vi "Test Save TGA (Memory).vi"(8 "error in (no error)":errorcluster) -> (0 "error out":errorcluster, 3 "Pass?":bool)   [LabVIEW 2020]
uses:
  <vilib>/picture/picture.llb/imagedata.ctl
  G-Image/Image IO/Polymorphic VIs/Save PNG Image (Memory).vi/23d07dd8-0246-46c8-8885-479f1b0fb2b3.vi
  G-Image/Private/Result To Error.vi
  G-Image/Private/Get Image Data.vi
  G-Image/Private/ARGB To RGBA.vi
  G-Image/Private/Depth To Number Channels.vi
  G-Image/Image Processing/Indexed Color To True Color Image.vi
  <vilib>/Utility/error.llb/Error Cluster From Error Code.vi
  G-Image/G-Image.lvlib
  G-Image/Image IO/Polymorphic VIs/Save TGA Image (Memory).vi
  G-Image/Image IO/Polymorphic VIs/Load Image (Memory).vi
panel:
  out "Array":cluster{string, "new picture":picture}[](array[cluster])
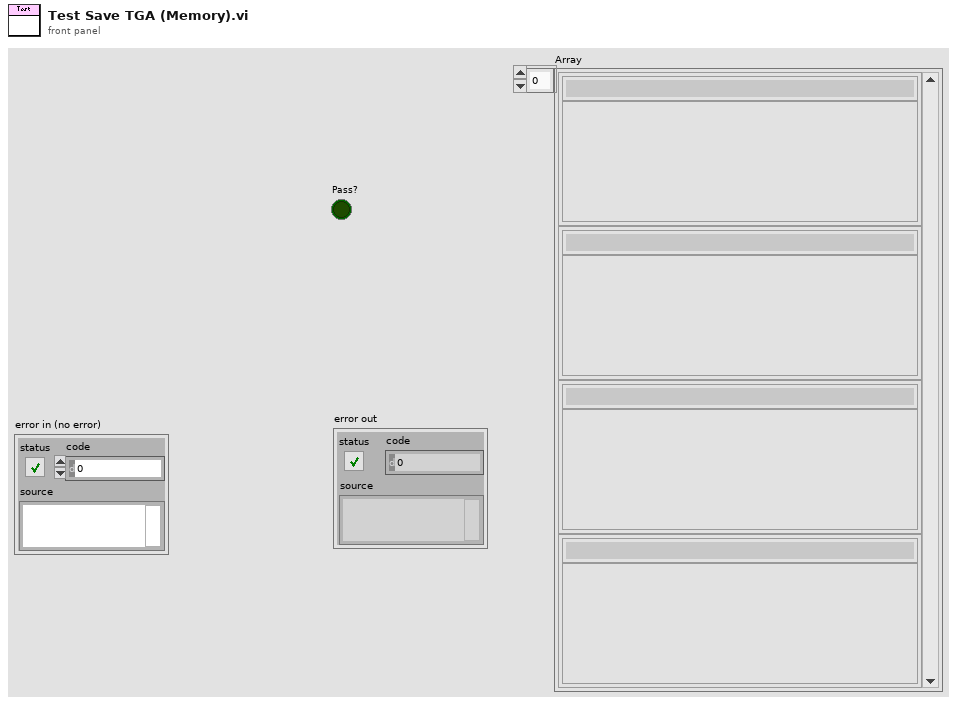
[diagram p1: front panel]
types:
  T1 = typedef "imagedata.ctl" = cluster{"image type":i32, "image depth":i32, "image":u8[], "mask":u8[], "colors":u32[], "Rectangle":cluster{"left":i16, "top":i16, "right":i16, "bottom":i16}}
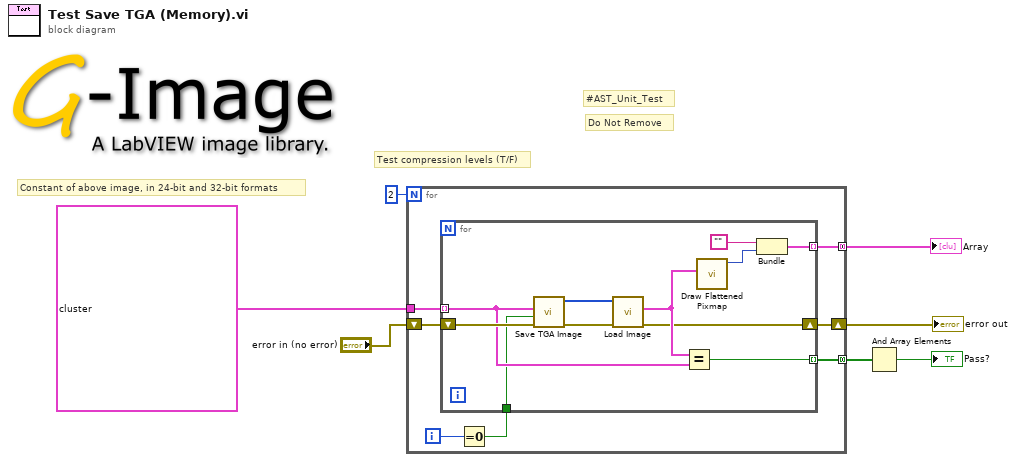
[diagram p0: block diagram]
diagram:
  # "Test compression levels (T/F)"
  # "Constant of above image, in 24-bit and 32-bit formats"
  # "Do Not Remove"
  # "#AST_Unit_Test"
  n1 = for {
    N: 2 -> [_]
    tunnel: [w13] -> w6 mode=concatenating
    tunnel: [w11] -> w4 mode=concatenating
    tunnel: T1[] [{"image type"=0, "image depth"=24, "image"=array[115500 elements], "mask"=[], "colors"=[], "Rectangle"={"left"=0, "top"=0, "right"=350, "bottom"=110}}, {"image type"=0, "image depth"=32, "image"=array[154000 elements], "mask"=array[4840 elements], "colors"=[], "Rectangle"={"left"=0, "top"=0, "right"=350, "bottom"=110}}] ("Array 2") -> [w10]
    shift-right: [w12] -> w5
    shift-left: "error in (no error)" -> [w14]
    i -> [w9]
    n2 = Equal To 0?(x=w9) -> (x = 0?=w8:bool)
    n3 = for {
      tunnel: w10 -> [w22] mode=indexing
      shift-right: [w16] -> w12
      shift-left: w14 -> [w25]
      tunnel: [w21] -> w11 mode=indexing
      tunnel: [w18] -> w13 mode=indexing
      tunnel: w8 -> [w15]
      n4 = call-poly "Save TGA Image.vi"("error in (no error)"=w25, "Compress (T)"=w15, "Image"=w22) -> ("error out"=w23:errorcluster, "Encoded Image"=w24:u8[])  [unwired: 7 in]
      n5 = call-poly "Load Image.vi"("error in (no error)"=w23, "Encoded Image"=w24) -> ("error out"=w16:errorcluster, "Image"=w20:T1)  [unwired: 8 in]
      n6 = Equal?(x=w20, y=w22) -> (x = y?=w21:bool)
      n7 = call <vilib>:"Draw Flattened Pixmap.vi"("image data"=w20) -> ("new picture"=w19:picture)  [unwired: 8 in]
      n8 = Bundle("", "new picture"=w19) -> (w18:cluster{string, "new picture":picture})  [unwired: 1 in]
    }
  }
  "error out" <- w5
  "Array" <- w6
  n9 = And Array Elements(Boolean array=w4) -> (logical AND=→"Pass?":bool)
